vi "Strafe Correct.vi"(6 "Reset":bool, 7 "Max Steer":dbl=0.05 format="%#_13g", 9 "Steer In":dbl, 11 "X In":dbl) -> (1 "Correction Active":bool, 3 "Angle Target":dbl)   [LabVIEW 2013]
uses:
  Common Code/Change Detect Boolean.vi
  <vilib>/Rock Robotics/WPI/Gyro/WPI_GyroRefNum Registry Get.vi
  Robot Global Data.vi
  <vilib>/Rock Robotics/WPI/Gyro/WPI_GyroGetAngle.vi
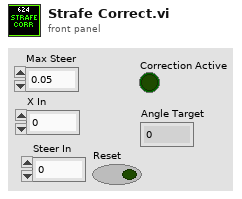
[diagram p1: front panel]
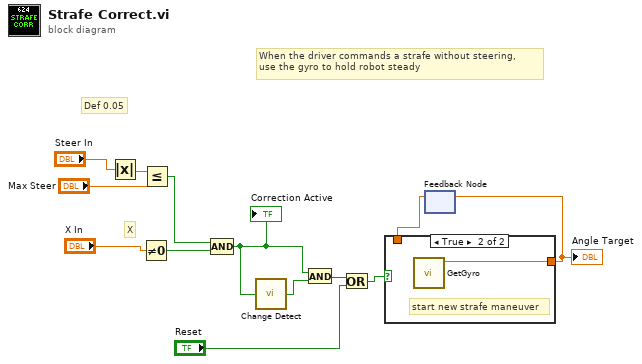
[diagram p0: block diagram]
diagram:
  # "When the driver commands a strafe without steering, \nuse the gyro to hold robot steady"
  # "Def 0.05"
  # "X"
  n1 = Absolute Value(x="Steer In") -> (abs(x)=w7:dbl)
  n2 = Not Equal To 0?(x="X In") -> (x != 0?=w11:bool)
  n3 = Less Or Equal?(x=w7, y="Max Steer") -> (x <= y?=w10:bool)
  n4 = Compound Arithmetic op=AND(w10, w11) -> (w12:bool)
  "Correction Active" <- w12
  n5 = call-poly "Change Detect.vi"("In"=w12) -> ("Changed?"=w6:bool)
  n6 = And(x=w12, y=w6) -> (x .and. y?=w3:bool)
  n7 = Or(x=w3, y="Reset") -> (x .or. y?=w2:bool)
  n8 = feedback #1() -> (w5:dbl)  [unwired: 1 in]
  n9 = case shown="True" w2 {
    tunnel: [w14 w15] -> w13
    tunnel: w5 -> [w14 _]
    frame False {
    }
    frame True {
      # "start new strafe maneuver"
      n10 = call "GetGyro.vi"() -> ("Angle"=w15:dbl)  [unwired: 9 in, 2 out]
    }
  }
  "Angle Target" <- w13
  n11 = feedback-in #1(w13) -> ()
